vi "c2f_subroutine.vi"() -> ()   [LabVIEW 2018]
panel:
  out "Numeric 2":dbl
  in  "Numeric":dbl
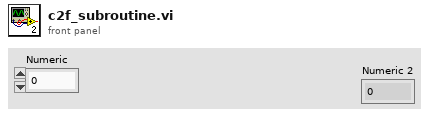
[diagram p1: front panel]
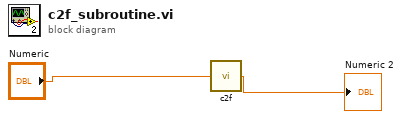
[diagram p0: block diagram]
diagram:
  n1 = call "c2f.vi"("degree\nc"="Numeric") -> ("degree f"=→"Numeric 2":dbl)
